vi "THzTime_SPEED_control_for Varying Gap_170202.vi"(1 "ESP300 Axis":i8=1, 2 "ESP300 Address":string="1", 4 "Lockin Address":string="12") -> ()   [LabVIEW 2010]
panel:
  in  "?":bool
  out "Current Round":i32=160
  out "Current Gap (um)":u32=100
  in  "Initial Gap (um)":u32=100
  out "error out":errorcluster
  in  "Number of Gap":u32=8
  in  "Number of Avg":u32=20
  in  "Gap Increase (um)":u32=25
  in  "Step Increase (um)":u32=5
  in  "error in (no error)":errorcluster
  in  "MCS System Locator":string="usb:id:1441320285"
  out "Y position":dbl=-5.0 format="%#.3p"
  out "X position":dbl=-5.0 format="%#.3p"
  out "Power meter":dbl format="%#.3p"
  in  "Save File Name":string="vg_"
  in  "Launch server?":bool
  in  "Authorize?":bool=TRUE
  in  "CONEX-PSD9 Instrument Key 2":string="CONEX-PSD (A6ULD73M)"
  in  "Interdelay (ms)":dbl=20.0
  in  "pre delay(ms)":dbl=300.0
  out "Lock-in Y-Channel":dbl=4.3656e-11 format="%#.3p"
  out "Lock-in X-Channel":dbl=7.4579e-11 format="%#.3p"
  out "THz Time-domain Signal Wave":cluster{"x-axis":sgl[], "y-axis":dbl[]}(graph)
  in  "Autosave Directory for Long-term Average Scan":path=path "D:/taianh/Measurement Data/170204 Variable Gap"
  out "Phase":cluster{"f0":dbl, "df":dbl, "magnitude":dbl[]}(graph)={"f0"=0.0, "df"=0.06507592594933881, "magnitude"=[3.141592653589793, -1.563981552163864, -1.5571668438336175, -1.5503521373100477, -1.5435373619231623, -1.5367225827486255, -1.5299078782588478, -1.5230931805187462, -1.5162783985320043, -1.5094636060480255, -1.5026489147948086, -1.4958342422583941, -1.4890194421952987, -1.4822046111427627, -1.4753899637937211, -1.4685753945582622, -1.4617605411726111, -1.454945467115905, -1.4481314583274683, -1.441314576382688, -1.4345012286676666, -1.4276868557476325, -1.4208718735514754, -1.4140569396453, -1.4072423683751119, -1.4004277910367307, -1.3936128985025549, -1.386797978849283, -1.3799833566456998, -1.373168773226224, -1.3663538542500753, -1.359538848904758, -1.352724229364266, -1.3459097286270965, -1.339094595112584, -1.3322789076126678, -1.3254637091948183, -1.3186531936899168, -1.3118372422788473, -1.3050226131102856, -1.2982070793768714, -1.2913917920447162, -1.2845772624648915, -1.277762762204734, -1.270947717506615, -1.2641326184103518, -1.2573180169231317, -1.2505034948644955, -1.2436884424450692, -1.2368732299663592, -1.2300585699720918, -1.2232440675852208, -1.2164286360209091, -1.2096123661912292, -1.2027964050355402, -1.195974895539818, -1.189178397443028, -1.1823606383311571, -1.1755437791599932, -1.1687278209089436, -1.1619132214672625, -1.1550987729465967, -1.1482835750820348, -1.1414683055085004, -1.134653759336068, -1.1278393804484965, -1.1210243265598674, -1.114209074692465, -1.107394589314625, -1.100580429299379, -1.0937653189421317, -1.086949596704172, -1.0801353756634129, -1.0733240324616224, -1.0665029085698474, -1.0596930502426054, -1.0528767729514794, -1.0460609984482023, -1.0392468554754253, -1.032432803279029, -1.0256176643776334, -1.0188023428057813, -1.0119879150315052, -1.0051737157133354, -0.9983586701678092, -0.9915433321339258, -0.9847288927264921, -0.9779148665463462, -0.9710997565255559, -0.9642839283949937, -0.9574696533501699, -0.9506575507998744, -0.9438449375562198, -0.9370292173204897, -0.9302115521244033, -0.9233952502579016, -0.9165812550650828, -0.9097674221761308, -0.9029522020758755, -0.8961367021991297, -0.8893222839155874, -0.8825081818030063, -0.8756930807987916, -0.8688775804104422, -0.8620630779822331, -0.8552490609689009, -0.8484338233526774, -0.8416176924954415, -0.8348029684002318, -0.8279896632530197, -0.8211711377523842, -0.8143804128251431, -0.8075498577764583, -0.8007315922198427, -0.7939173177957869, -0.7871035205670177, -0.7802881110102817, -0.7734723660656454, -0.766657931786088, -0.7598439527266077, -0.7530288734598071, -0.7462133215452416, -0.7393988986893498, -0.7325851127034775, -0.725770120775291, -0.7189542807418903, -0.7121401208880314, -0.7053279969678171, -0.6985143906268976, -0.6916907019947772, -0.6848791051745625, -0.6780624807149682, -0.6712494761645633, -0.6644365141966455, -0.6576213508443927, -0.6508056049567682, -0.6439912898131427, -0.6371775048164067, -0.6303624689276216, -0.6235468188831239, -0.6167323383602411, -0.6099185569047552, -0.6031034792249897, -0.5962873840245416, -0.5894727831267856, -0.5826597902186963, -0.5758442016626426, -0.5690179304728984, -0.5622248046980518, -0.5553997570398271, -0.5485859250430141, -0.5417728319616035, -0.5349573338824054, -0.5281412119351773, -0.5213267735530945, -0.5145130410636565, -0.5076979892546252, -0.5008822358886232, -0.4940677304537473, -0.4872540518395547, -0.48043910065948403, -0.4736231094057407, -0.4668086581986669, -0.45999597507174916, -0.45318142612722295, -0.44636254885905535, -0.4395632154710582, -0.4327296722942684, -0.4259181592573783, -0.41910616907268344, -0.41229092687371804, -0.4054747602314405, -0.3986604016407296, -0.3918468529133744, -0.38503187281341866, -0.37821605504476324, -0.3714015015472507, -0.3645878533273339, -0.357772921644116, -0.35095685683993877, -0.34414222871173816, -0.337329275019072, -0.33051447498644404, -0.3236958494383334, -0.3168769787447932, -0.31006271626731, -0.30325241098305467, -0.2964408165818027, -0.2896253295691716, -0.282808766612551, -0.2759942230137747, -0.26918064028800864, -0.2623655422018306, -0.25554946704013803, -0.2487346348566173, -0.24192074280154888, -0.23510551298393056, -0.22828896652290387, -0.22147357062301362, -0.21465945670671097, -0.20784291533280455, -0.2010211607879454, -0.19419173409451812, -0.18750826776253274, -0.18060475018937508, -0.1737863089177277, -0.16696788265335244, -0.16014960511049656, -0.1533341703667902, -0.1465201808322328, -0.13970481868838724, -0.13288850797546714, -0.1260735530693798, -0.11925972647131047, -0.11244472236425294, -0.10562850300390052, -0.09881355697461726, -0.09200022791389079, -0.08518537627577642, -0.07836762056451586, -0.07155110438710488, -0.06474590952842135, -0.05792379631265704, -0.051114070048657416, -0.04429803697363414, -0.037480748554359684, -0.03066603603030896, -0.023852672601392136, -0.017037737680903553, -0.010221648516429812, -0.003406831888749156]}
  in  "OK Button":bool
  out "Data Type":string="outp ? 1"
  in  "Enum":enum16{"X", "Y", "Abs"}(ring)
  in  "Draw":bool
  in  "Exit Program":bool
  out "Amplitude":cluster{"f0":dbl, "df":dbl, "magnitude":dbl[]}(graph)={"f0"=0.0, "df"=0.06507592594933881, "magnitude"=[17.350000741424893, 0.5188112757865829, 0.25941165281266815, 0.17294780094575565, 0.12971788381968372, 0.10378153327129408, 0.08649197213181646, 0.074143440154787, 0.06488304726600498, 0.057681408441869954, 0.051920901950551296, 0.04720849814345019, 0.04328216798588641, 0.03996050340478469, 0.03711393755647227, 0.034647460723669525, 0.03248980365470768, 0.03058645327286037, 0.028895013559795558, 0.027382079308321698, 0.026020833815437048, 0.0247896342783373, 0.023670727298899057, 0.022649461065755095, 0.021713641120819725, 0.020853020933033702, 0.02005891773219348, 0.01932393518436375, 0.018641744445596325, 0.01800689099104938, 0.01741463720584481, 0.016860854049706653, 0.01634193955704272, 0.01585473342715652, 0.015396434627410182, 0.014964551039633149, 0.014556876770354653, 0.014171535550895514, 0.013806605783497712, 0.013460660772823397, 0.013132217592157455, 0.012819990854004166, 0.012522834449679214, 0.012239704549013328, 0.011969638453304263, 0.011711759290703337, 0.011465277911510339, 0.011229473789866834, 0.011003675874948894, 0.010787265114695719, 0.010579682878099975, 0.01038041937853304, 0.010188992287904864, 0.010004946886649744, 0.009827878799988964, 0.009657512491304325, 0.009493083171555835, 0.009334838570576227, 0.009182164732025875, 0.009034799446660078, 0.008892494653195207, 0.00875501068181151, 0.008622107908152312, 0.008493561924011708, 0.008369174229812454, 0.008248760209953902, 0.008132135715764289, 0.008019124531984336, 0.007909571421449615, 0.0078033350529348585, 0.007700270627759322, 0.007600232495885576, 0.0075030950120080165, 0.007408757906005036, 0.007317094715829411, 0.007228042511681897, 0.007141436932128122, 0.0070571913801245525, 0.006975231194500595, 0.0068954784033766975, 0.006817843003548391, 0.006742239596870925, 0.006668599459681427, 0.0065968592206603355, 0.006526947726877214, 0.006458793837021259, 0.006392340135822829, 0.006327536896296744, 0.006264325711307569, 0.006202642454648159, 0.006142437765091036, 0.006083682554307576, 0.006026400936325213, 0.005970291321188627, 0.0059155901711074495, 0.005862129550304197, 0.005809894242382125, 0.005758856373016857, 0.005708971642497486, 0.005660197612994174, 0.005612506631397871, 0.005565874525779105, 0.005520267135793496, 0.005475647953420541, 0.005431992096333163, 0.005389280847075778, 0.0053474857544928344, 0.005306571389837766, 0.0052665148145175445, 0.005227309133154267, 0.005188945703989573, 0.005151328758109325, 0.005114535401807436, 0.005078467019429951, 0.005043138010209762, 0.005008539288771296, 0.004974643412119527, 0.004941424168555739, 0.0049088700705315885, 0.004876972790987731, 0.004845713174877077, 0.0048150686655785225, 0.004785027507349614, 0.004755583757923823, 0.004726721683712459, 0.004698418187086736, 0.004670661360667103, 0.004643453072673571, 0.004616786852172034, 0.004590598708376208, 0.004564985611937733, 0.004539804723832213, 0.0045151152301117015, 0.004490913754721776, 0.004467179242307117, 0.0044438922815692745, 0.004421048818912292, 0.004398648109886207, 0.004376678112582228, 0.004355122724384199, 0.004333976260728626, 0.004313238914412172, 0.004292901367526543, 0.00427294691087429, 0.004253369411806125, 0.0042341760927948075, 0.00421536872203828, 0.00419695778654655, 0.00417868436002762, 0.0041609505993381365, 0.004143523880837004, 0.004126442207235193, 0.004109691401962572, 0.004093256399874347, 0.0040771376033164, 0.004061338710391739, 0.004045851588932044, 0.004030663433612093, 0.004015771597416693, 0.004001179463017942, 0.0039868811470594396, 0.0039728631823495834, 0.003959121727215751, 0.003945664780263116, 0.003932492107346465, 0.0039195845616949825, 0.003906949926020683, 0.0038945176822510166, 0.0038823763153433112, 0.0038705056338847812, 0.003858888091354034, 0.0038475091019830525, 0.0038363711929929357, 0.0038254806229226605, 0.0038148314314515844, 0.0038044124970287013, 0.0037942227525273363, 0.0037842674327425007, 0.003774542798280462, 0.0037650373939210027, 0.003755748698212389, 0.0037466852698777816, 0.0037378473112138874, 0.0037292159772247917, 0.0037207535600292368, 0.0037125948294360355, 0.003704566577964215, 0.0036967744256863467, 0.0036891894468663766, 0.0036817965267886446, 0.003674599736468162, 0.0036676072546924982, 0.0036608145519772795, 0.0036542114480478355, 0.0036477977937526365, 0.003641580079682178, 0.0036355561214748357, 0.0036297159138716627, 0.003624057880295388, 0.0036185912302863464, 0.003613317714711174, 0.0036082235703284297, 0.003603303579798647, 0.003598392737034303, 0.0035939366658638127, 0.003589573714184675, 0.003585382461651676, 0.0035813537417174403, 0.0035774946695606704, 0.003573815650318573, 0.003570313426669526, 0.0035669784547252663, 0.0035638112007018046, 0.0035608191074655614, 0.0035580011736887373, 0.0035553483853115317, 0.003552859607825008, 0.003550544103063903, 0.0035484039678675534, 0.003546426283740626, 0.0035446027466432286, 0.003542972599004621, 0.003541425591290441, 0.0035401337211347205, 0.0035389977177766323, 0.003538011623571554, 0.003537184488143226, 0.0035365283434483086, 0.003536040719781041, 0.0035357123349429543, 0.0035355440292435527]}
  in  "Short term \nAverage#":i8=1
  in  "Step":sgl=0.005 min=0 max=10000 format="%.3f"
  in  "End Position":sgl=-18.5 min=-75 max=75 format="%#.3f"
  in  "Start Position":sgl=-16.2 min=-75 max=75 format="%#.3f"
  # "Data"
  # "Auto-offset"
  # "Start Position (mm)"
  # "End Position (mm)"
  # "Step (mm)"
  # "Point Avg"
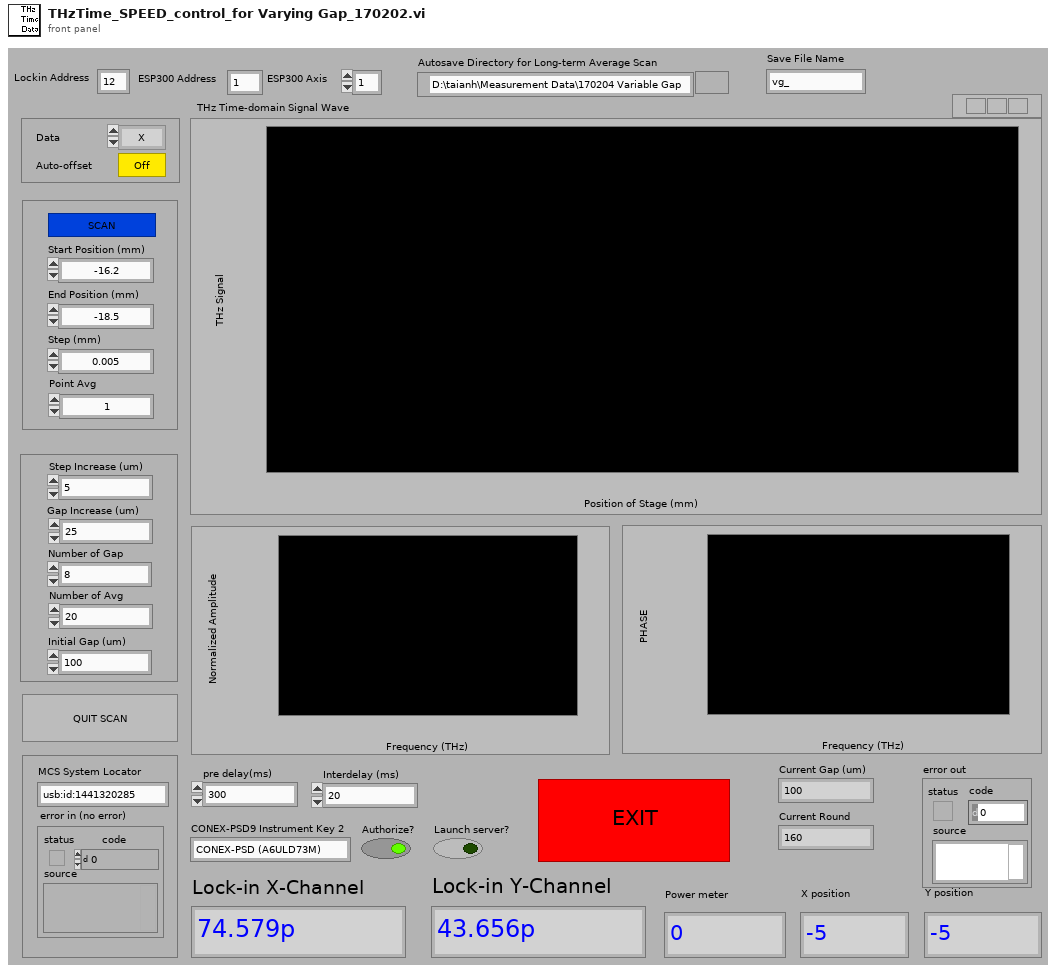
[diagram p1: front panel]
types:
  T1 = cluster{"ConexPSD Reference":refnum<k24>, "error out":errorcluster, "Component ID":i32}
  T2 = cluster{"System Index Out":u32, "error out":errorcluster}
  T3 = cluster{"Step Number":i32, "Step":sgl, "Start Position":sgl, "Time-out":i32, "Lockin Address":string, "Short term \nAverage#":i8, i32, "ESP300 Axis":i8, "Value":string, "pre delay(ms)":dbl, "Interdelay (ms)":dbl, "Autosave Directory for Long-term Average Scan":path, cluster{"ConexPSD Reference":refnum<k24>, "error out":errorcluster, "Component ID":i32}}
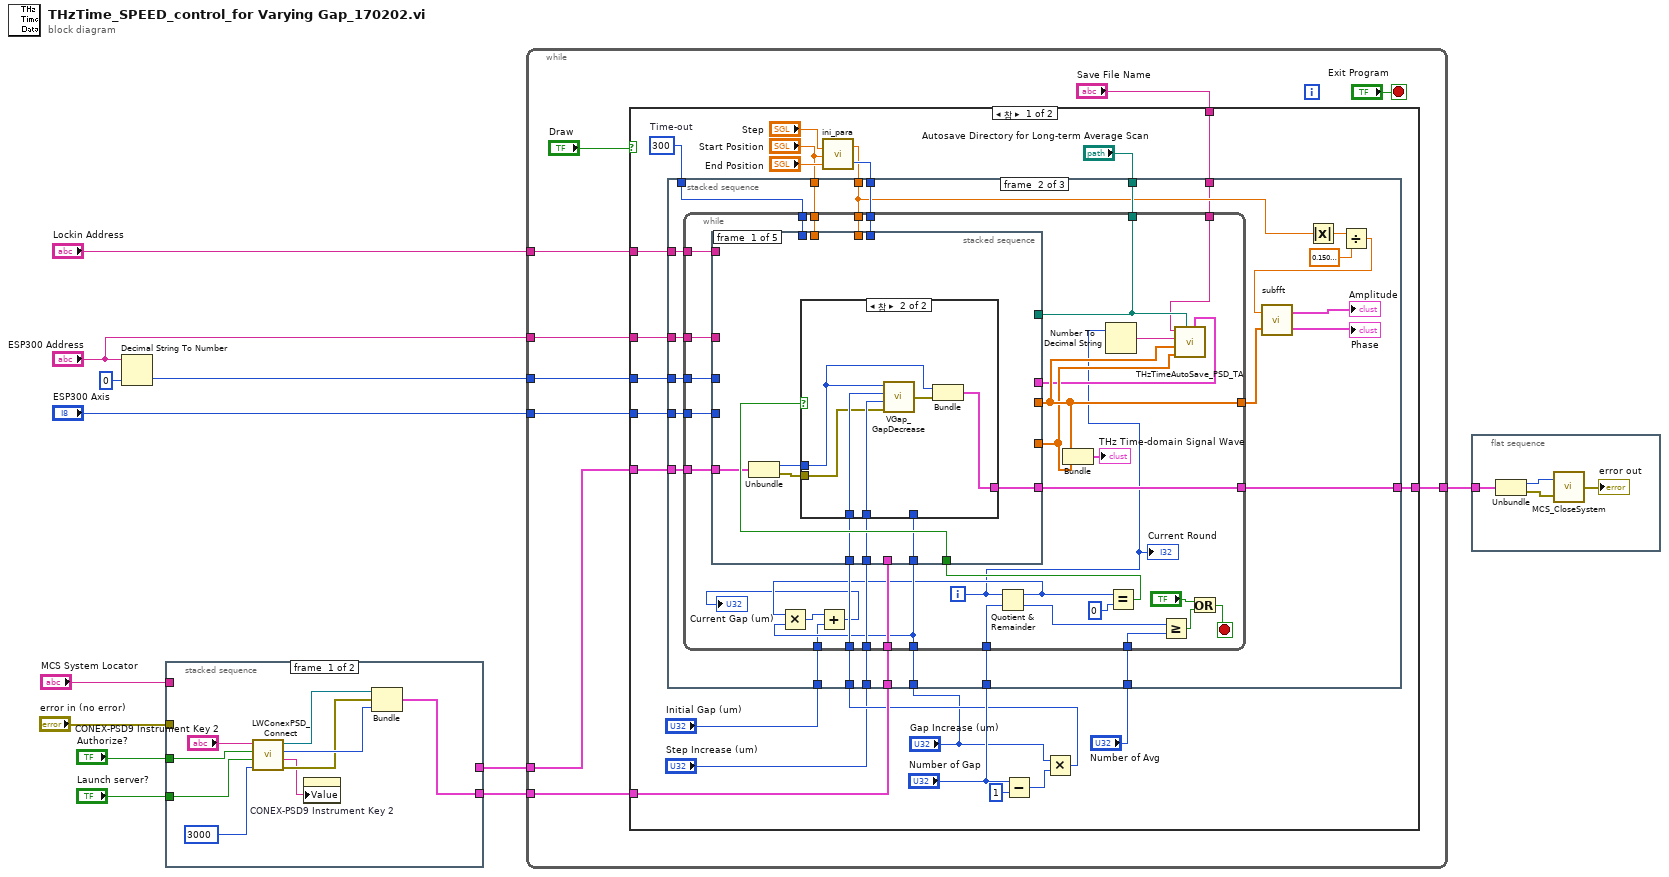
[diagram p0: block diagram]
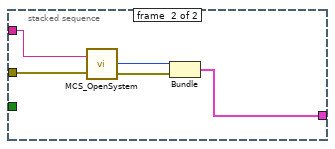
[diagram p2: hidden frame]
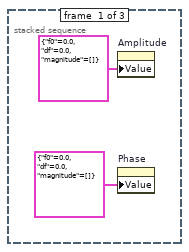
[diagram p3: hidden frame]
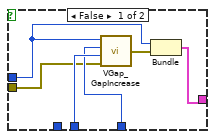
[diagram p4: hidden frame]
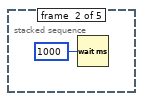
[diagram p5: hidden frame]
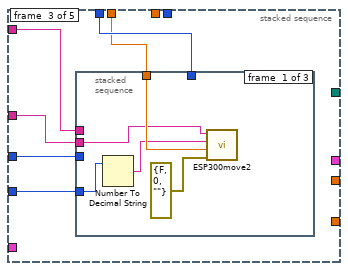
[diagram p6: hidden frame]
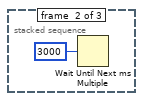
[diagram p7: hidden frame]
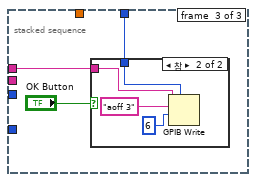
[diagram p8: hidden frame]
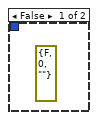
[diagram p9: hidden frame]
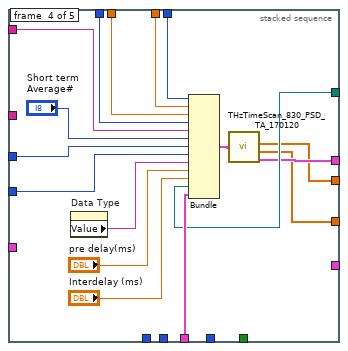
[diagram p10: hidden frame]
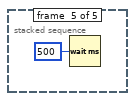
[diagram p11: hidden frame]
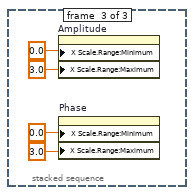
[diagram p12: hidden frame]
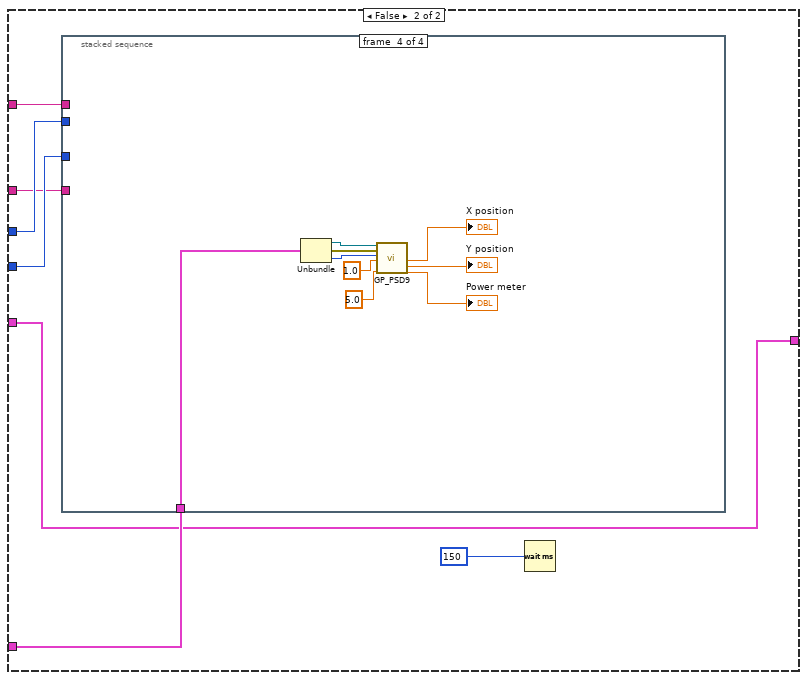
[diagram p13: hidden frame]
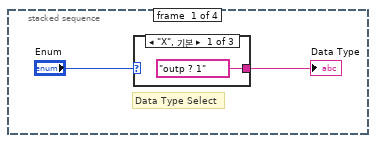
[diagram p14: hidden frame]
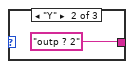
[diagram p15: hidden frame]
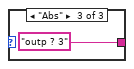
[diagram p16: hidden frame]
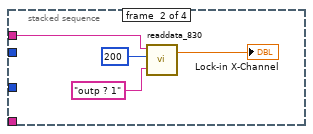
[diagram p17: hidden frame]
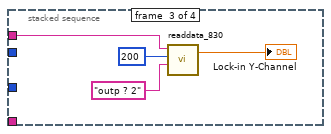
[diagram p18: hidden frame]
diagram:
  n1 = Decimal String To Number(string="ESP300 Address", default (0L)=0 ("default (0 I32)")) -> (number=w10:i32)  [unwired: 1 in, 1 out]
  n2 = stacked-sequence {
    tunnel: "Authorize?" -> [w15 _]
    tunnel: [w14 _] -> w5
    tunnel: "Launch server?" -> [w13 _]
    tunnel: "MCS System Locator" -> [_ w26]
    tunnel: "error in (no error)" -> [_ w25]
    tunnel: [_ w22] -> w2
    frame #0 {
      n3 = call "LWConexPSD_Connect.vi"("DiscoverTimeout (10000 msec)"=3000, "Launch server? (True)"=w13, "Authorize? (True)"=w15, "Instrument Key"="CONEX-PSD9 Instrument Key 2") -> ("error out"=w19:errorcluster, "Instrument Key out"=w17:string, "Component ID"=w20:i32, "ConexPSD Reference"=w18:refnum<k24>)
      n4 = property on="CONEX-PSD9 Instrument Key 2" class="Str"("Value"=w17) -> ()  [unwired: 2 in, 2 out]
      n5 = Bundle("ConexPSD Reference"=w18, "error out"=w19, "Component ID"=w20) -> (w14:T1)  [unwired: 1 in]
    }
    frame #1 {
      n6 = call "MCS_OpenSystem.vi"("error in (no error)"=w25, "MCS System Locator"=w26) -> ("error out"=w23:errorcluster, "System Index Out"=w24:u32)
      n7 = Bundle("System Index Out"=w24, "error out"=w23) -> (w22:T2)  [unwired: 1 in]
    }
  }
  n8 = while {
    tunnel: "ESP300 Axis" -> [w34]
    tunnel: "Lockin Address" -> [w33]
    tunnel: w10 -> [w32]
    tunnel: "ESP300 Address" -> [w31]
    tunnel: w5 -> [w30]
    tunnel: w2 -> [w28]
    tunnel: [w27] -> w1
    stop <- "Exit Program" stop-if-true
    n9 = case shown="참" "Draw" {
      tunnel: w33 -> [w59 w187]
      tunnel: w34 -> [w58 w189]
      tunnel: w32 -> [w57 w188]
      tunnel: w31 -> [w49 w185]
      tunnel: w30 -> [w48 w184]
      tunnel: "Save File Name" -> [w47 _]
      tunnel: w28 -> [w46 w183]
      tunnel: [w38 w183] -> w27
      frame True {
        w56 = 300  # Time-out
        n10 = call "ini_para.vi"("End Position"="End Position", "Start Position"="Start Position", "Step"="Step") -> ("Step Number"=w53:i32, "Step"=w52:sgl)
        n11 = Subtract(x="Number of Gap", y=u32 1) -> (x-y=w43:u32)
        n12 = Multiply(x="Gap Increase (um)", y=w43) -> (x*y=w42:u32)
        n13 = stacked-sequence {
          tunnel: w59 -> [_ w86 _]
          tunnel: w56 -> [_ w85 _]
          tunnel: w58 -> [_ w84 _]
          tunnel: w57 -> [_ w83 _]
          tunnel: w53 -> [_ w81 _]
          tunnel: w52 -> [_ w75 _]
          tunnel: "Start Position" -> [_ w82 _]
          tunnel: "Autosave Directory for Long-term Average Scan" -> [_ w80 _]
          tunnel: w49 -> [_ w73 _]
          tunnel: w48 -> [_ w72 _]
          tunnel: w47 -> [_ w71 _]
          tunnel: "Number of Gap" -> [_ w69 _]
          tunnel: w46 -> [_ w68 _]
          tunnel: w42 -> [_ w67 _]
          tunnel: "Step Increase (um)" -> [_ w66 _]
          tunnel: "Gap Increase (um)" -> [_ w65 _]
          tunnel: "Number of Avg" -> [_ w64 _]
          tunnel: [_ w63 _] -> w38
          tunnel: "Initial Gap (um)" -> [_ w62 _]
          frame #0 {
            n14 = property on="Amplitude" class="WFGraph (엄격한)"("Value"=cluster{"f0":dbl, "df":dbl, "magnitude":dbl[]} {"f0"=0.0, "df"=0.0, "magnitude"=[]} ("Spectrum")) -> ()  [unwired: 2 in, 2 out]
            n15 = property on="Phase" class="WFGraph (엄격한)"("Value"=cluster{"f0":dbl, "df":dbl, "magnitude":dbl[]} {"f0"=0.0, "df"=0.0, "magnitude"=[]} ("Spectrum")) -> ()  [unwired: 2 in, 2 out]
          }
          frame #1 {
            n16 = while {
              tunnel: w85 -> [w119]
              tunnel: w86 -> [w120]
              tunnel: w84 -> [w118]
              tunnel: w83 -> [w117]
              tunnel: w82 -> [w116]
              tunnel: w75 -> [w115]
              tunnel: w81 -> [w114]
              tunnel: w80 -> [w107]
              tunnel: [w109] -> w70
              tunnel: w73 -> [w112]
              tunnel: w72 -> [w111]
              tunnel: w71 -> [w106]
              tunnel: w69 -> [w104]
              tunnel: w68 -> [w101]
              tunnel: w67 -> [w97]
              tunnel: w66 -> [w100]
              tunnel: w65 -> [w96]
              tunnel: w64 -> [w99]
              tunnel: [w98] -> w63
              tunnel: w62 -> [w92]
              i -> [w94]
              stop <- w87 stop-if-true
              n17 = Quotient & Remainder(x=w94, y=w104) -> (x-y*floor(x/y)=w95:u32, floor(x/y)=w93:u32)
              n18 = Multiply(x=w95, y=w96) -> (x*y=w91:u32)
              n19 = Add(x=w91, y=w92) -> (x+y=→"Current Gap (um)":u32)
              n20 = Number To Decimal String(number=w94) -> (decimal integer string=w110:string)  [unwired: 1 in]
              n21 = Equal?(x=w95, y=u32 0) -> (x = y?=w102:bool)
              n22 = stacked-sequence {
                tunnel: w120 -> [_ _ w147 w173 _]
                tunnel: w119 -> [_ _ w146 w174 _]
                tunnel: w118 -> [_ _ w145 w170 _]
                tunnel: w117 -> [_ _ w144 w171 _]
                tunnel: w116 -> [_ _ w143 w175 _]
                tunnel: w115 -> [_ _ _ w176 _]
                tunnel: w114 -> [_ _ _ w177 _]
                tunnel: [_ _ _ w162 _] -> w109
                tunnel: [_ _ _ w161 _] -> w108
                tunnel: w112 -> [_ _ w142 _ _]
                tunnel: w107 -> [_ _ _ w165 _]
                tunnel: w111 -> [_ _ _ w166 _]
                tunnel: [_ _ _ w163 _] -> w105
                tunnel: w102 -> [w128 _ _ _ _]
                tunnel: w101 -> [w124 _ _ _ _]
                tunnel: w97 -> [w127 _ _ _ _]
                tunnel: w100 -> [w126 _ _ _ _]
                tunnel: w96 -> [w125 _ _ _ _]
                tunnel: [w121 _ _ _ _] -> w98
                frame #0 {
                  n23 = Unbundle(w124) -> ("System Index Out"=w122:u32, "error out"=w123:errorcluster)
                  n24 = case shown="참" w128 {
                    tunnel: w127 -> [_ w140]
                    tunnel: w126 -> [w134 w139]
                    tunnel: w125 -> [w133 _]
                    tunnel: w122 -> [w130 w136]
                    tunnel: w123 -> [w132 w138]
                    tunnel: [w129 w135] -> w121
                    frame False {
                      n25 = call "VGap_GapIncrease.vi"("error in (no error)"=w132, "Step Increase (um)"=w134, "Gap Increase (um)"=w133, "System Index In"=w130) -> ("error out"=w131:errorcluster)
                      n26 = Bundle("System Index Out"=w130, "error out"=w131) -> (w129:T2)  [unwired: 1 in]
                    }
                    frame True {
                      n27 = call "VGap_GapDecrease.vi"("error in (no error)"=w138, "Step Decrease (um)"=w139, "Gap Decrease (um)"=w140, "System Index In"=w136) -> ("error out"=w137:errorcluster)
                      n28 = Bundle("System Index Out"=w136, "error out"=w137) -> (w135:T2)  [unwired: 1 in]
                    }
                  }
                }
                frame #1 {
                  n29 = Wait (ms)(milliseconds to wait=u32 1000 ("대기 시간(ms)")) -> ()  [unwired: 1 out]
                }
                frame #2 {
                  n30 = stacked-sequence {
                    tunnel: w147 -> [_ _ w155]
                    tunnel: w146 -> [_ _ w154]
                    tunnel: w145 -> [w149 _ _]
                    tunnel: w144 -> [_ _ _]
                    tunnel: w143 -> [w152 _ _]
                    tunnel: w142 -> [w150 _ _]
                    frame #0 {
                      n31 = Number To Decimal String(number=w149) -> (decimal integer string=w148:string)  [unwired: 1 in]
                      n32 = call "ESP300move2.vi"("ESP300 Address"=w150, "ESP300 Channel"=w148, "Target"=w152, "error in (no error) 2"=errorcluster {"status"=FALSE, "code"=0, "source"=""}) -> ()  [unwired: 6 in, 1 out]
                    }
                    frame #1 {
                      n33 = Wait Until Next ms Multiple(millisecond multiple=3000) -> ()  [unwired: 1 out]
                    }
                    frame #2 {
                      n34 = case shown="참" "OK Button" {
                        tunnel: w155 -> [_ w160]
                        tunnel: w154 -> [_ w158]
                        frame False {
                          (unwired) errorcluster {"status"=FALSE, "code"=0, "source"=""} ("error in")
                        }
                        frame True {
                          n35 = GPIB Write(0:w160, 1:"aoff 3" ("data"), 2:i16 6 ("mode (0)"), 4:w158) -> ()  [unwired: 1 in, 2 out]
                        }
                      }
                    }
                  }
                }
                frame #3 {
                  n36 = property on="Data Type" class="Str"() -> ("Value"=w169:string)  [unwired: 2 in, 2 out]
                  n37 = Bundle("Step Number"=w177, "Step"=w176, "Start Position"=w175, "Time-out"=w174, "Lockin Address"=w173, "Short term \nAverage#"="Short term \nAverage#", w171, "ESP300 Axis"=w170, "Value"=w169, "pre delay(ms)"="pre delay(ms)", "Interdelay (ms)"="Interdelay (ms)", "Autosave Directory for Long-term Average Scan"=w165, w166) -> (w164:T3)  [unwired: 1 in]
                  n38 = call "THzTimeScan_830_PSD_TA_170120.vi"("input"=w164) -> ("x-axis"=w162:sgl[], "y-axis"=w161:dbl[], "ext. out"=w163:cluster{dbl[], dbl[], dbl[], dbl[], string[]})  [unwired: 1 out]
                }
                frame #4 {
                  n39 = Wait (ms)(milliseconds to wait=u32 500) -> ()  [unwired: 1 out]
                }
              }
              n40 = Bundle("x-axis"=w109, "y-axis"=w108) -> (→"THz Time-domain Signal Wave":cluster{"x-axis":sgl[], "y-axis":dbl[]})  [unwired: 1 in]
              n41 = Greater Or Equal?(x=w93, y=w99) -> (x >= y?=w88:bool)
              n42 = call "THzTimeAutoSave_PSD_TA.vi"("ext. out"=w105, "Autosave Directory for Long-term Average Scan"=w107, "y-axis"=w108, "x-axis"=w109, "String"=w110, "SaveFile name"=w106) -> ()  [unwired: 4 in]
              n43 = Or(x="?", y=w88) -> (x .or. y?=w87:bool)
              "Current Round" <- w94
            }
            n44 = Absolute Value(x=w75) -> (abs(x)=w76:sgl)
            n45 = Divide(x=w76, y=sgl 0.15) -> (x/y=w74:sgl)
            n46 = call "subfft.vi"("y-signal"=w70, "time step"=w74) -> ("Phase"=→"Phase":cluster{"f0":dbl, "df":dbl, "real part":dbl[]}, "Amplitude"=→"Amplitude":cluster{"f0":dbl, "df":dbl, "real part":dbl[]})
          }
          frame #2 {
            n47 = property on="Amplitude" class="WFGraph (엄격한)"("X Scale.Range:Minimum"=0.0 ("X Scale.Range:Maximum"), "X Scale.Range:Maximum"=3.0) -> ()  [unwired: 2 in, 2 out]
            n48 = property on="Phase" class="WFGraph (엄격한)"("X Scale.Range:Minimum"=0.0, "X Scale.Range:Maximum"=3.0) -> ()  [unwired: 2 in, 2 out]
          }
        }
      }
      frame False {
        n49 = stacked-sequence {
          tunnel: w189 -> [_ _ _ _]
          tunnel: w188 -> [_ _ _ _]
          tunnel: w187 -> [_ w198 w202 _]
          tunnel: w185 -> [_ _ _ _]
          tunnel: w184 -> [_ _ _ w203]
          frame #0 {
            # "Data Type Select"
            n50 = case shown="\"X\", 기본" "Enum" {
              tunnel: ["outp ? 1" "outp ? 2" "outp ? 3"] -> w191
              frame "X", Default {
              }
              frame "Y" {
              }
              frame "Abs" {
              }
            }
            "Data Type" <- w191
          }
          frame #1 {
            n51 = call "readdata_830.vi"("Command"="outp ? 1", "timeout"=200, "Lockin Address"=w198) -> ("Data"=→"Lock-in X-Channel":dbl)  [unwired: 1 in, 1 out]
          }
          frame #2 {
            n52 = call "readdata_830.vi"("Command"="outp ? 2", "timeout"=200, "Lockin Address"=w202) -> ("Data"=→"Lock-in Y-Channel":dbl)  [unwired: 1 in, 1 out]
          }
          frame #3 {
            n53 = Unbundle(w203) -> ("ConexPSD Reference"=w211:refnum<k24>, "error out"=w210:errorcluster, "Component ID"=w209:i32)
            n54 = call "GP_PSD9.vi"("ConexPSD Reference"=w211, "error out"=w210, "Component ID"=w209, "Adress"=1.0 ("shot average"), "shot average"=5.0) -> ("PositionX"=→"X position":dbl, "PositionY"=→"Y position":dbl, "LaserPower"=→"Power meter":dbl)  [unwired: 8 in, 4 out]
          }
        }
        n55 = Wait (ms)(milliseconds to wait=u32 150) -> ()  [unwired: 1 out]
      }
    }
  }
  n56 = flat-sequence {
    tunnel: w1 -> [w215]
    frame #0 {
      n57 = Unbundle(w215) -> ("System Index Out"=w214:u32, "error out"=w213:errorcluster)
      n58 = call "MCS_CloseSystem.vi"("error in (no error)"=w213, "System Index In"=w214) -> ("error out"=→"error out":errorcluster)
    }
  }
